vi "Make_Mirror_Pattern_V1.vi"(0 "Mirror Modes In":T1, 2 "Flat On?":bool, 7 "Flat File In":dbl[](array[numeric]), 11 "Mirror Modes Array":dbl[][](array[numeric]), 13 "Amplitude Scale Factor":dbl=5500.0 format="%#_13g") -> (8 "Pixel Value U (-1 to 1)":dbl[](array[numeric]))   [LabVIEW 2016]
uses:
  Controls/MirrorModes.ctl
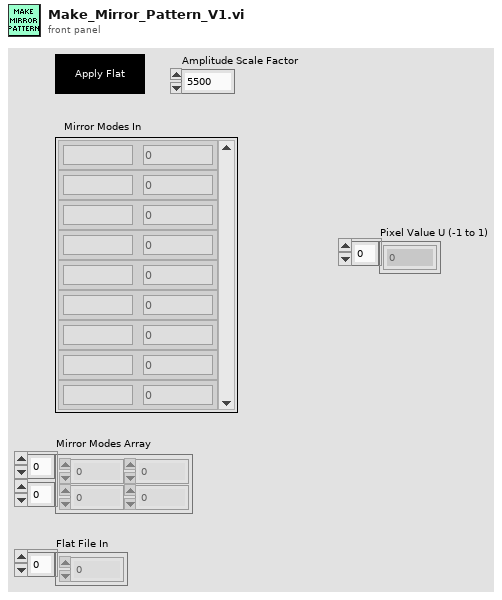
[diagram p1: front panel]
types:
  T1 = typedef "MirrorModes.ctl" = cluster{"Mode":string, "Amplitude":dbl}[]
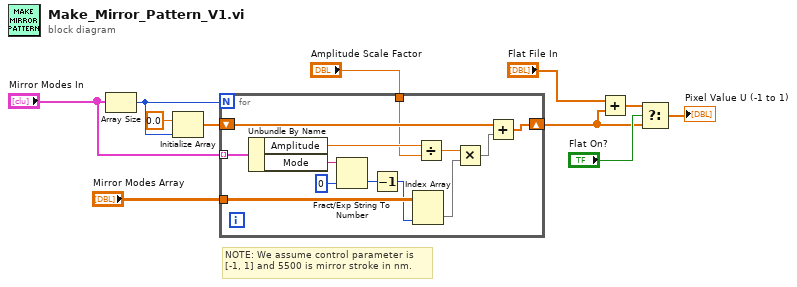
[diagram p0: block diagram]
diagram:
  # "NOTE: We assume control parameter is\n[-1, 1] and 5500 is mirror stroke in nm."
  n1 = Array Size(array="Mirror Modes In") -> (size(s)=w10:i32)
  n2 = Initialize Array(0.0 ("element"), w10) -> (w4:dbl[])
  n3 = for {
    N: w10 -> [_]
    tunnel: "Mirror Modes In" -> [w24] mode=indexing
    shift-right: [w17] -> w5
    shift-left: w4 -> [w18]
    tunnel: "Mirror Modes Array" -> [w20]
    tunnel: "Amplitude Scale Factor" -> [w12]
    n4 = Unbundle By Name(w24) -> ("Amplitude"=w13:dbl, "Mode"=w22:string)
    n5 = Fract/Exp String To Number(string=w22, default (0 dbl)=0) -> (number=w21:i32)  [unwired: 2 in, 1 out]
    n6 = Decrement(x=w21) -> (x-1=w19:i32)
    n7 = Index Array(array=w20, index (col)=w19) -> (element=w14:dbl[])  [unwired: 1 in]
    n8 = Divide(x=w13, y=w12) -> (x/y=w15:dbl)
    n9 = Multiply(x=w15, y=w14) -> (x*y=w16:dbl[])
    n10 = Add(x=w18, y=w16) -> (x+y=w17:dbl[])
  }
  n11 = Add(x="Flat File In", y=w5) -> (x+y=w9:dbl[])
  n12 = Select(t=w9, s="Flat On?", f=w5) -> (s? t:f=→"Pixel Value U (-1 to 1)":dbl[])
